vi "CSMOMgr-Delete CSMO.vi"(8 "Error In":errorcluster caption="error in (no error)", 10 "Queue Name":string, 11 "CSMOMgr":T1) -> (0 "error out":errorcluster, 3 "CSMOMgr Out":T1)   [LabVIEW 2017, in "Communicable State Machine.lvlib"]
uses:
  Communicable State Machine.lvlib
  Def-CSMOMgr.ctl
  FGV-BroadcastRegistry/Operation-BroadcastRegistry.ctl
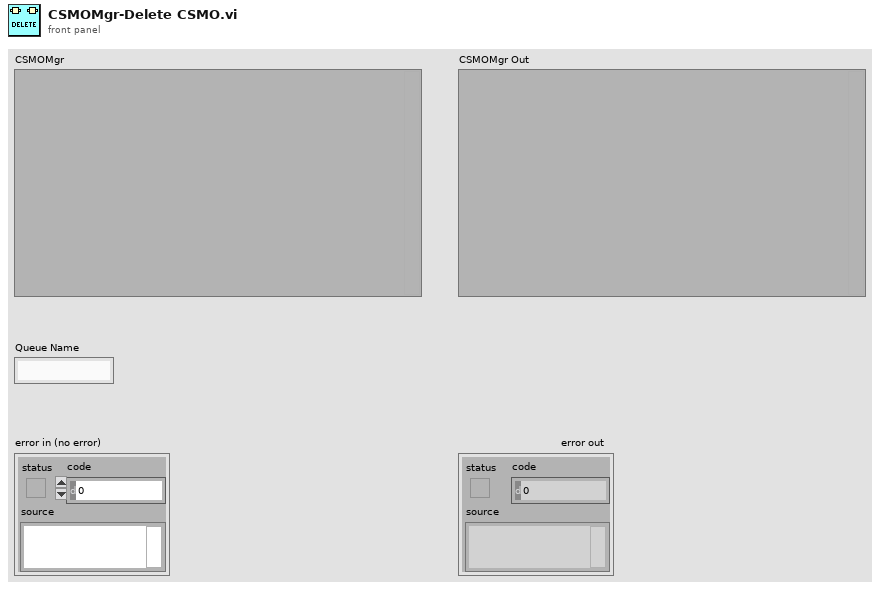
[diagram p1: front panel]
types:
  T1 = typedef "Communicable State Machine.lvlib/Def-CSMOMgr.ctl" = variant
  T2 = typedef "Communicable State Machine.lvlib/_CSMObj.ctl" = cluster{"info":T3, "Refs":T5}
  T3 = typedef "Communicable State Machine.lvlib/_CSMObj-Info.ctl" = cluster{"Module Name":string, "Requested Name":string, "Group Name":string, "Mode":T4, "Allowed Messages":string[]}
  T4 = typedef "Communicable State Machine.lvlib/_CSM_MODE.ctl" = enum16{"Not Exist", "Stand Alone", "CSM", "Worker", "Worker Agent", "Chain Node", "Chain"}
  T5 = typedef "Communicable State Machine.lvlib/_CSMObj-Refs.ctl" = cluster{"WatchDogQ":refnum<queue>, "CSMDataDVR":refnum<data-value>, "Queue":T6, "GroupDataDVR":refnum<data-value>, "TagMap":refnum<data-value>, "ExitEvent":refnum<user-event>, "NewStateEvent":refnum<user-event>, "StatusChangeEvent":refnum<user-event>}
  T6 = typedef "Communicable State Machine.lvlib/Priority Queue.ctl" = cluster{"HPriorityQ":refnum<queue>, "LowPriorityQ":refnum<queue>}
  T7 = typedef "Communicable State Machine.lvlib/Operation-BroadcastRegistry.ctl" = enum16{"Delete Source Module", "Delete Target Module", "Remove Module", "Register", "Unregister", "Check", "List Status", "List Entries", "List Status Of Source", "Drop"}
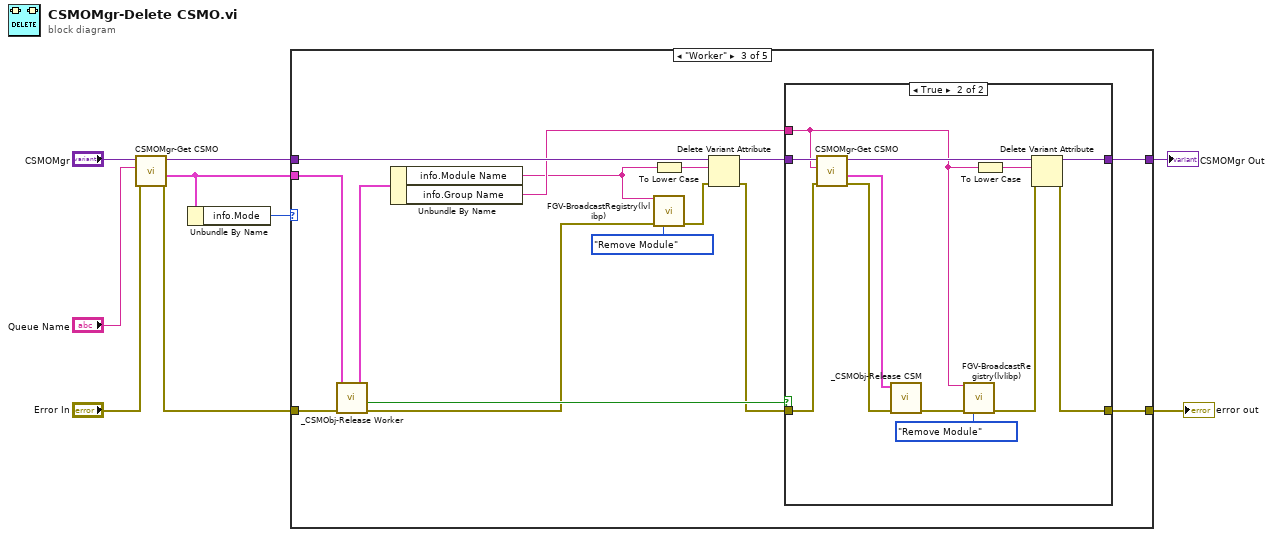
[diagram p0: block diagram]
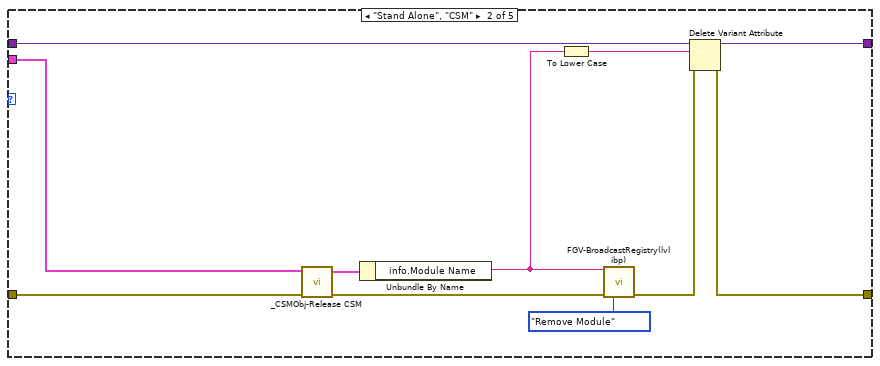
[diagram p3: hidden frame]
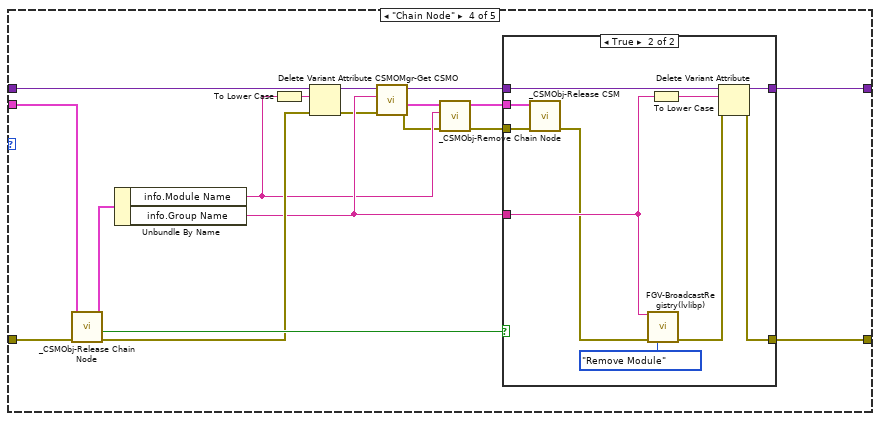
[diagram p5: hidden frame]
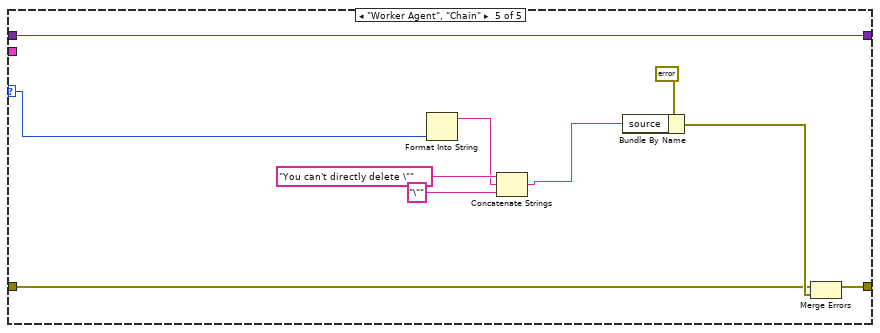
[diagram p7: hidden frame]
diagram:
  n1 = call "CSMOMgr-Get CSMO.vi"("Error In"="Error In", "Queue Name"="Queue Name", "CSMOMgr"="CSMOMgr") -> ("error out"=w9:errorcluster, "Values"=w7:T2, "CSMOMgr Out"=w8:T1)  [unwired: 5 in, 1 out]
  n2 = Unbundle By Name(w7) -> ("info.Mode"=w6:T4)
  n3 = case shown="\"Worker\"" w6 {
    selector: w6 -> [_ _ _ _ w82]
    tunnel: [w11 w22 w37 w69 w91] -> w2
    tunnel: [w10 w21 w36 w68 w85] -> w1
    tunnel: w7 -> [_ w20 w35 w67 _]
    tunnel: w9 -> [w10 w19 w33 w65 w84]
    tunnel: w8 -> [w11 w18 w32 w61 w91]
    frame "Not Exist", Default {
    }
    frame "Stand Alone", "CSM" {
      n4 = call "_CSMObj-Release CSM.vi"("Error In"=w19, "CSMQ In"=w20) -> ("error out"=w16:errorcluster, "CSMQ Out"=w17:T2)  [unwired: 7 in, 1 out]
      n5 = Unbundle By Name(w17) -> ("info.Module Name"=w14:string)
      n6 = To Lower Case(string=w14) -> (all lower case string=w12:string)
      n7 = call "FGV-BroadcastRegistry(lvlibp).vi"("Source"=w14, "Error In"=w16, "Operation"=Operation-BroadcastRegistry."Remove Module") -> ("error out"=w15:errorcluster)  [unwired: 11 in, 1 out]
      n8 = Delete Variant Attribute(4:w15, 6:w12, 7:w18) -> (0:w21:errorcluster, 3:w22:variant)  [unwired: 1 out]
    }
    frame "Worker" {
      n9 = call "_CSMObj-Release Worker.vi"("Error In"=w33, "CSMQ In"=w35) -> ("error out"=w25:errorcluster, "Group Release?"=w34:bool, "CSMQ Out"=w29:T2)  [unwired: 7 in]
      n10 = Unbundle By Name(w29) -> ("info.Module Name"=w24:string, "info.Group Name"=w28:string)
      n11 = To Lower Case(string=w24) -> (all lower case string=w23:string)
      n12 = call "FGV-BroadcastRegistry(lvlibp).vi"("Source"=w24, "Error In"=w25, "Operation"=Operation-BroadcastRegistry."Remove Module") -> ("error out"=w26:errorcluster)  [unwired: 11 in, 1 out]
      n13 = Delete Variant Attribute(4:w26, 6:w23, 7:w32) -> (0:w30:errorcluster, 3:w31:variant)  [unwired: 1 out]
      n14 = case shown="True" w34 {
        tunnel: w28 -> [_ w43]
        tunnel: w31 -> [w39 w45]
        tunnel: [w39 w50] -> w37
        tunnel: w30 -> [w38 w42]
        tunnel: [w38 w48] -> w36
        frame False {
        }
        frame True {
          n15 = call "CSMOMgr-Get CSMO.vi"("Error In"=w42, "Queue Name"=w43, "CSMOMgr"=w45) -> ("error out"=w40:errorcluster, "Values"=w41:T2, "CSMOMgr Out"=w44:T1)  [unwired: 5 in, 1 out]
          n16 = call "_CSMObj-Release CSM.vi"("Error In"=w40, "CSMQ In"=w41) -> ("error out"=w46:errorcluster)  [unwired: 7 in, 2 out]
          n17 = call "FGV-BroadcastRegistry(lvlibp).vi"("Source"=w43, "Error In"=w46, "Operation"=Operation-BroadcastRegistry."Remove Module") -> ("error out"=w49:errorcluster)  [unwired: 11 in, 1 out]
          n18 = To Lower Case(string=w43) -> (all lower case string=w47:string)
          n19 = Delete Variant Attribute(4:w49, 6:w47, 7:w44) -> (0:w48:errorcluster, 3:w50:variant)  [unwired: 1 out]
        }
      }
    }
    frame "Chain Node" {
      n20 = call "_CSMObj-Release Chain Node.vi"("Error In"=w65, "CSMQ In"=w67) -> ("error out"=w64:errorcluster, "Group Release?"=w66:bool, "CSMQ Out"=w63:T2)  [unwired: 7 in]
      n21 = Unbundle By Name(w63) -> ("info.Module Name"=w56:string, "info.Group Name"=w62:string)
      n22 = To Lower Case(string=w56) -> (all lower case string=w53:string)
      n23 = Delete Variant Attribute(4:w64, 6:w53, 7:w61) -> (0:w58:errorcluster, 3:w60:variant)  [unwired: 1 out]
      n24 = call "CSMOMgr-Get CSMO.vi"("Error In"=w58, "Queue Name"=w62, "CSMOMgr"=w60) -> ("error out"=w55:errorcluster, "Values"=w57:T2, "CSMOMgr Out"=w59:T1)  [unwired: 5 in, 1 out]
      n25 = call "_CSMObj-Remove Chain Node.vi"("Error In"=w55, "Requested Name"=w56, "CSMObj In"=w57) -> ("error out"=w54:errorcluster, "CSMObj Out"=w52:T2)  [unwired: 7 in]
      n26 = case shown="True" w66 {
        tunnel: w62 -> [_ w78]
        tunnel: w59 -> [w71 w80]
        tunnel: [w71 w79] -> w69
        tunnel: w54 -> [w70 w73]
        tunnel: [w70 w76] -> w68
        tunnel: w52 -> [_ w74]
        frame False {
        }
        frame True {
          n27 = call "_CSMObj-Release CSM.vi"("Error In"=w73, "CSMQ In"=w74) -> ("error out"=w72:errorcluster)  [unwired: 7 in, 2 out]
          n28 = call "FGV-BroadcastRegistry(lvlibp).vi"("Source"=w78, "Error In"=w72, "Operation"=Operation-BroadcastRegistry."Remove Module") -> ("error out"=w77:errorcluster)  [unwired: 11 in, 1 out]
          n29 = To Lower Case(string=w78) -> (all lower case string=w75:string)
          n30 = Delete Variant Attribute(4:w77, 6:w75, 7:w80) -> (0:w76:errorcluster, 3:w79:variant)  [unwired: 1 out]
        }
      }
    }
    frame "Worker Agent", "Chain" {
      n31 = Format Into String(w82) -> (resulting string=w83:string)  [unwired: 3 in, 1 out]
      n32 = Concatenate Strings("You can't directly delete \"" ("source"), w83, "\"" ("source")) -> (w87:string)
      n33 = Bundle By Name(cluster=errorcluster {"status"=TRUE, "code"=-1, "source"=""} ("error out"), "source"=w87) -> (w86:errorcluster)
      n34 = Merge Errors(w84, w86) -> (w85:errorcluster)
    }
  }
  "error out" <- w1
  "CSMOMgr Out" <- w2
